vi "Report filter for report breakdown summery.vi"() -> ()   [LabVIEW 2017]
panel:
  in  "Report filter":string
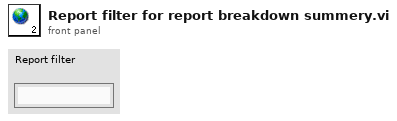
[diagram p1: front panel]
diagram:
